vi "Check Result.vi"(10 "actual temperature":dbl[unit]=273.15, 11 "thermal test":refnum<class "Thermal Test.lvclass">) -> (2 "pass?":bool)   [LabVIEW 2023, in "Thermal Test.lvclass"]
uses:
  Thermal Test.lvclass
  Thermal Test.lvclass/Thermal Test.ctl
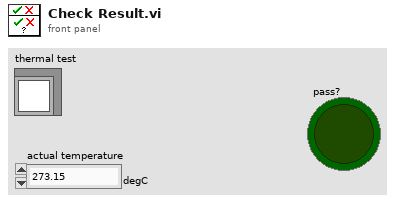
[diagram p1: front panel]
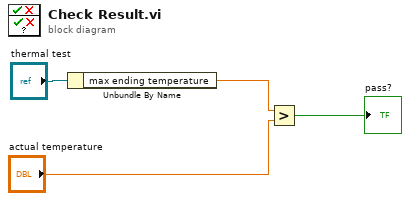
[diagram p0: block diagram]
diagram:
  n1 = Unbundle By Name("thermal test") -> ("max ending temperature"=w3:dbl[unit])
  n2 = Greater?(x=w3, y="actual temperature") -> (0:→"pass?":bool)
